vi "CommCheck_v4.0.vi"(5 "error in":errorcluster) -> (0 "Oracle\nComm. Success":bool, 1 "Vision\nComm. Success":bool, 2 "Barcode\nComm. Success":bool, 3 "COMM SUCCESS":bool, 4 "error out":errorcluster)   [LabVIEW 2019]
panel:
  out "Vision IP":string
  out "Barcode IP":string
  out "Barcode Port":string
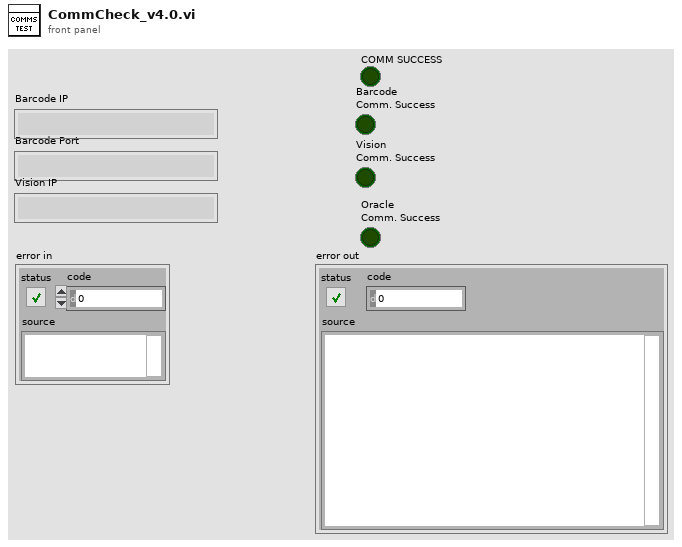
[diagram p1: front panel]
types:
  T1 = enum16{"Read Program", "Change Program", "Trigger 1", "Switch to Run Mode", "Blank"}
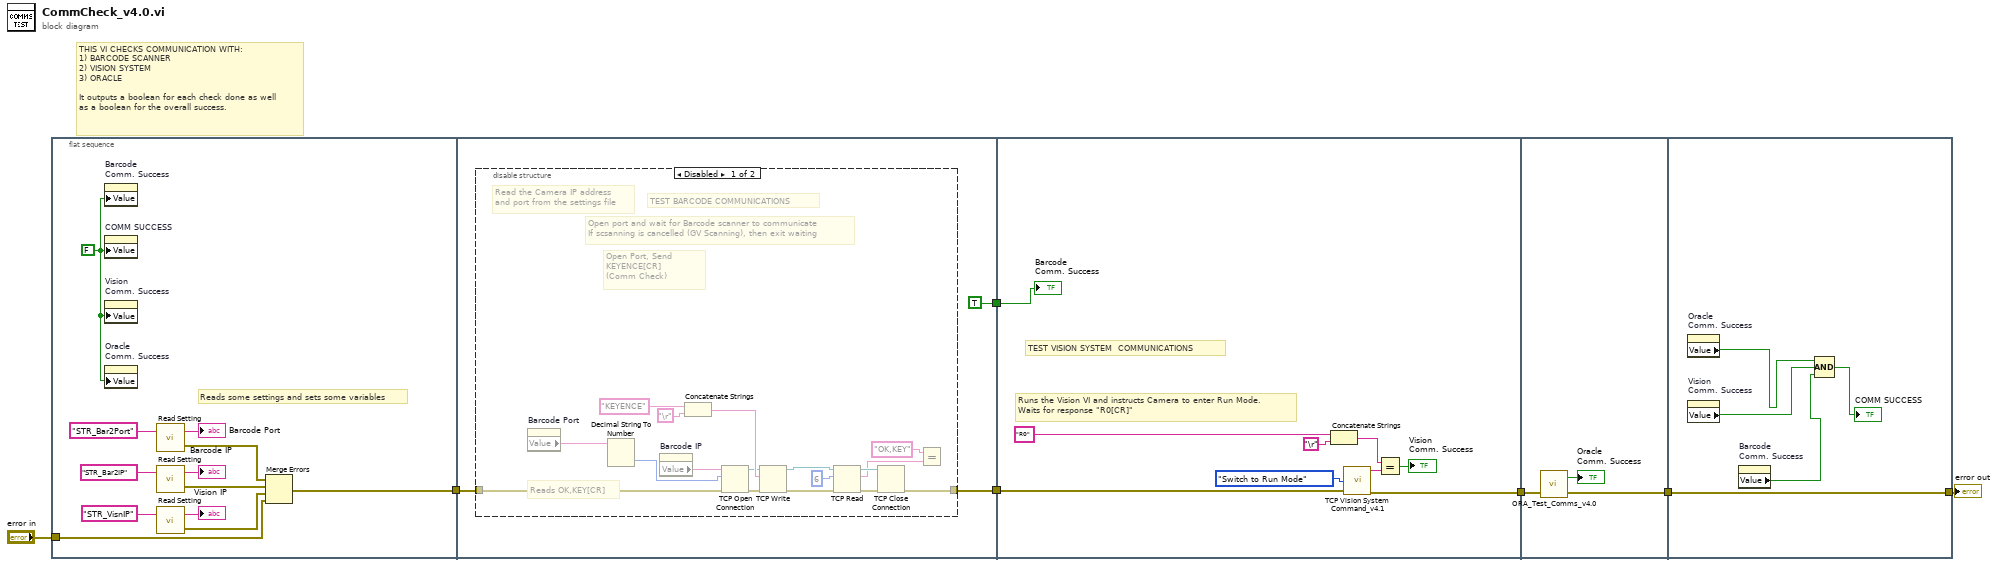
[diagram p0: block diagram]
diagram:
  # "THIS VI CHECKS COMMUNICATION WITH:\n1) BARCODE SCANNER\n2) VISION SYSTEM\n3) ORACLE\n\nIt outputs a boolean for each check done as well\nas a boolean for the overall success."
  n1 = flat-sequence {
    tunnel: "error in" -> [w9]
    tunnel: [w10] -> w5
    tunnel: [TRUE] -> w4
    tunnel: w5 -> [w22]
    tunnel: [w21] -> w3
    tunnel: w4 -> [w40]
    tunnel: w3 -> [w47]
    tunnel: [w44] -> w2
    tunnel: w2 -> [w50]
    tunnel: [w49] -> w1
    tunnel: [w56] -> w6
    tunnel: w1 -> [w56]
    frame #0 {
      w8 = FALSE ("Barcode\nComm. Success")
      # "Reads some settings and sets some variables"
      n2 = property on="Barcode\nComm. Success" class="Bool (strict)"("Value"=w8) -> ()  [unwired: 2 in, 2 out]
      n3 = property on="COMM SUCCESS" class="Bool (strict)"("Value"=w8) -> ()  [unwired: 2 in, 2 out]
      n4 = property on="Vision\nComm. Success" class="Bool (strict)"("Value"=w8) -> ()  [unwired: 2 in, 2 out]
      n5 = property on="Oracle\nComm. Success" class="Bool (strict)"("Value"=w8) -> ()  [unwired: 2 in, 2 out]
      n6 = call "Read Setting.vi"("Setting to read"="STR_Bar2Port") -> ("error out"=w11:errorcluster, "Setting Value"=→"Barcode Port":string)  [unwired: 1 in]
      n7 = call "Read Setting.vi"("Setting to read"="STR_Bar2IP") -> ("error out"=w13:errorcluster, "Setting Value"=→"Barcode IP":string)  [unwired: 1 in]
      n8 = call "Read Setting.vi"("Setting to read"="STR_VisnIP") -> ("error out"=w12:errorcluster, "Setting Value"=→"Vision IP":string)  [unwired: 1 in]
      n9 = Merge Errors(w11, w13, w12, w9) -> (w10:errorcluster)
    }
    frame #1 {
      n10 = disable-structure shown="Disabled" {
        disable-tunnel: w22 -> [w28 _]
        disable-tunnel: [w24 _] -> w21
        frame Disabled {
          # "TEST BARCODE COMMUNICATIONS"
          # "Open port and wait for Barcode scanner to communicate\nIf scsanning is cancelled (GV Scanning), then exit waiting"
          # "Reads OK,KEY[CR]"
          # "Open Port, Send KEYENCE[CR]\n(Comm Check)"
          # "Read the Camera IP address \nand port from the settings file"
          n11 = property on="Barcode Port" class="Str"() -> ("Value"=w27:string)  [unwired: 2 in, 2 out]
          n12 = Decimal String To Number(string=w27) -> (number=w34:i32)  [unwired: 2 in, 1 out]
          n13 = property on="Barcode IP" class="Str"() -> ("Value"=w26:string)  [unwired: 2 in, 2 out]
          n14 = Concatenate Strings("KEYENCE" ("data in"), "\r") -> (w33:string)
          n15 = TCP Open Connection(address=w26, remote port or service name=w34, error in (no error)=w28) -> (connection ID=w31:refnum<k5>, error out=w32:errorcluster)  [unwired: 2 in]
          n16 = TCP Write(connection ID=w31, data in=w33, error in (no error)=w32) -> (connection ID out=w35:refnum<k5>, error out=w36:errorcluster)  [unwired: 1 in, 1 out]
          n17 = TCP Read(connection ID=w35, bytes to read=6, error in (no error)=w36) -> (connection ID out=w37:refnum<k5>, data out=w23:string, error out=w38:errorcluster)  [unwired: 2 in]
          n18 = TCP Close Connection(connection ID=w37, error in (no error)=w38) -> (error out=w24:errorcluster)  [unwired: 1 in, 1 out]
          n19 = Equal?(x="OK,KEY" ("data in"), y=w23) -> ()  [unwired: 1 out]
        }
        frame Enabled {
        }
      }
    }
    frame #2 {
      # "Runs the Vision VI and instructs Camera to enter Run Mode.\nWaits for response \"R0[CR]\""
      # "TEST VISION SYSTEM  COMMUNICATIONS"
      n20 = Concatenate Strings("R0" ("data in"), "\r") -> (w41:string)
      n21 = call "TCP Vision System Command_v4.1.vi"("Enum"=T1."Switch to Run Mode", "error in (no error)"=w47) -> ("Response to Command"=w45:string, "error out"=w44:errorcluster)  [unwired: 1 in, 2 out]
      n22 = Equal?(x=w41, y=w45) -> (x = y?=→"Vision\nComm. Success":bool)
      "Barcode\nComm. Success" <- w40
    }
    frame #3 {
      n23 = call "ORA_Test_Comms_v4.0.vi"("error in (no error)"=w50) -> ("error out"=w49:errorcluster, "Successful Comm"=→"Oracle\nComm. Success":bool)  [unwired: 1 in]
    }
    frame #4 {
      n24 = property on="Oracle\nComm. Success" class="Bool (strict)"() -> ("Value"=w53:bool)  [unwired: 2 in, 2 out]
      n25 = property on="Vision\nComm. Success" class="Bool (strict)"() -> ("Value"=w54:bool)  [unwired: 2 in, 2 out]
      n26 = property on="Barcode\nComm. Success" class="Bool (strict)"() -> ("Value"=w55:bool)  [unwired: 2 in, 2 out]
      n27 = Compound Arithmetic op=AND(w53, w54, w55) -> (→"COMM SUCCESS":bool)
    }
  }
  "error out" <- w6
